vi "fo_ReadDICOMValues.vi"(11 "dataset":refnum<k24>) -> (1 "study date":string, 2 "study id":string, 3 "accession number":string)   [LabVIEW 2013, in "main.lvlib"]
uses:
  main.lvlib
  C:/Users/Simon/SkyDrive/LabView/2013/DM2020/bin/Dicom.dll
  bin/Dicom.dll
panel:
  in  "error in (no error)":errorcluster
  out "error out":errorcluster
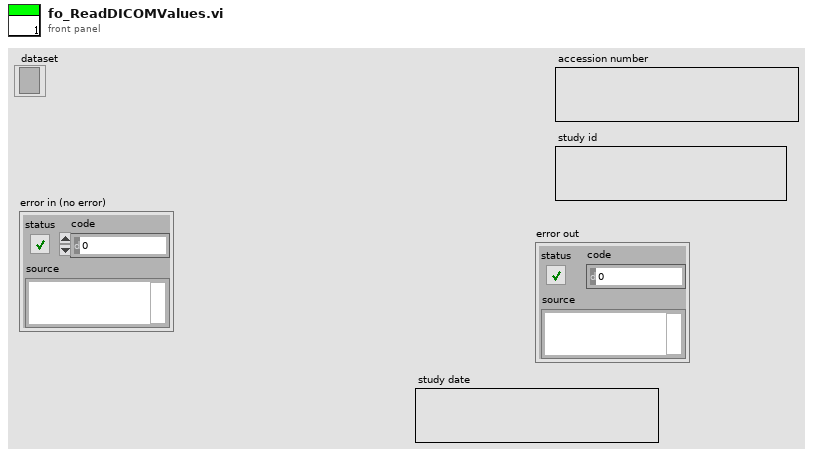
[diagram p1: front panel]
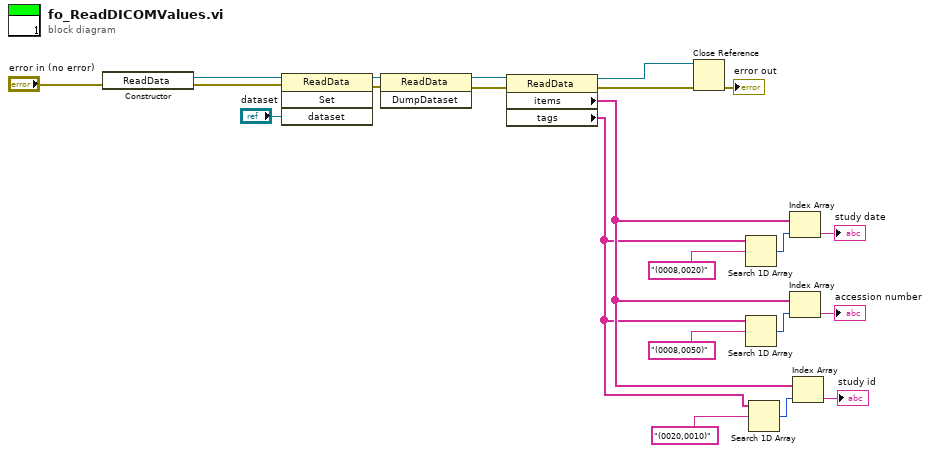
[diagram p0: block diagram]
diagram:
  n1 = constructor class="ReadData"(error in="error in (no error)") -> (reference out=w22:refnum<k24>, error out=w21:errorcluster)  [unwired: 2 in, 1 out]
  n2 = invoke class="ReadData" method="Set"(reference=w22, error in=w21, "dataset"="dataset") -> (reference out=w19:refnum<k24>, error out=w14:errorcluster)  [unwired: 1 in, 2 out]
  n3 = invoke class="ReadData" method="DumpDataset"(reference=w19, error in=w14) -> (reference out=w18:refnum<k24>, error out=w17:errorcluster)  [unwired: 1 in, 1 out]
  n4 = property class="ReadData"(reference=w18, error in=w17) -> (reference out=w16:refnum<k24>, error out=w15:errorcluster, "items"=w3:string[], "tags"=w2:string[])
  n5 = Close Reference(reference=w16, error in (no error)=w15) -> (error out=→"error out":errorcluster)
  n6 = Search 1D Array(1D array=w2, element="(0008,0020)") -> (index of element=w4:i32)  [unwired: 1 in]
  n7 = Search 1D Array(1D array=w2, element="(0008,0050)") -> (index of element=w12:i32)  [unwired: 1 in]
  n8 = Search 1D Array(1D array=w2, element="(0020,0010)") -> (index of element=w9:i32)  [unwired: 1 in]
  n9 = Index Array(array=w3, index=w4) -> (element=→"study date":string)
  n10 = Index Array(array=w3, index=w12) -> (element=→"accession number":string)
  n11 = Index Array(array=w3, index=w9) -> (element=→"study id":string)
